vi "Measurement UI.vi"() -> ()   [LabVIEW 2020, in "Waveform Measurement.lvlib"]
uses:
  Waveform Measurement.lvlib
  <vilib>/gRPC/Generated APIs/ni/protobuf/types/RPC Messages/ni_protobuf_types_DoubleAnalogWaveform_Flat.ctl
  <vilib>/gRPC/Generated APIs/ni/protobuf/types/RPC Messages/ni_protobuf_types_PrecisionTimestamp_Flat.ctl
  <vilib>/gRPC/Generated APIs/ni/protobuf/types/RPC Messages/ni_protobuf_types_DoubleAnalogWaveform_AttributesEntry_Flat.ctl
  <vilib>/gRPC/Generated APIs/ni/protobuf/types/RPC Messages/ni_protobuf_types_WaveformAttributeValue_Flat.ctl
  <vilib>/gRPC/Extensions/Extensions.lvlib
  <vilib>/gRPC/Generated APIs/ni/protobuf/types/ni.protobuf.types.lvlib
panel:
  in  "Signal Type":T1(ring)=enum."Sine"
  out "Waveform":T2
  out "Waveform Graph":waveform(dbl)(graph)
  in  "Offset":dbl
  in  "Sample Rate":u32=1000
  in  "Frequency":dbl=10.0
  in  "Amplitude":dbl=5.0
  in  "Number of Samples":u32=1000
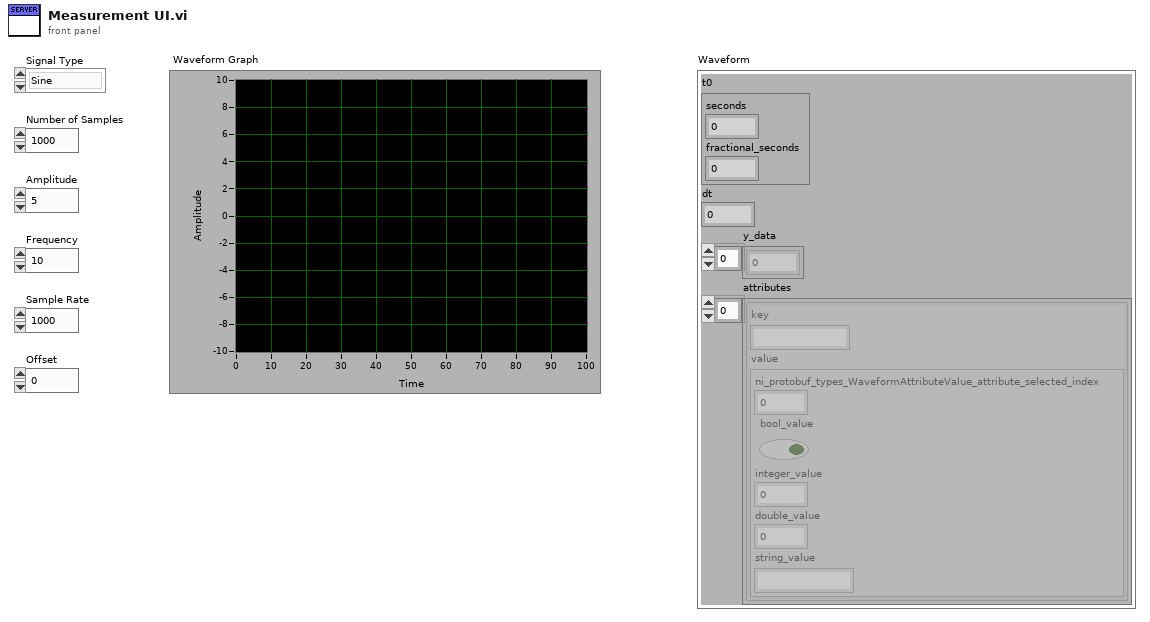
[diagram p1: front panel]
types:
  T1 = enum32{"None", "Sine", "Square", "Triangle", "Sawtooth"}
  T2 = typedef "ni.protobuf.types.lvlib/ni_protobuf_types_DoubleAnalogWaveform_Flat.ctl" = cluster{"t0":T3, "dt":dbl, "y_data":dbl[], "attributes":T4[]}
  T3 = typedef "ni.protobuf.types.lvlib/ni_protobuf_types_PrecisionTimestamp_Flat.ctl" = cluster{"seconds":i64, "fractional_seconds":u64}
  T4 = typedef "ni.protobuf.types.lvlib/ni_protobuf_types_DoubleAnalogWaveform_AttributesEntry_Flat.ctl" = cluster{"key":string, "value":T5}
  T5 = typedef "ni.protobuf.types.lvlib/ni_protobuf_types_WaveformAttributeValue_Flat.ctl" = cluster{"ni_protobuf_types_WaveformAttributeValue_attribute_selected_index":i32, "bool_value":bool, "integer_value":i32, "double_value":dbl, "string_value":string}
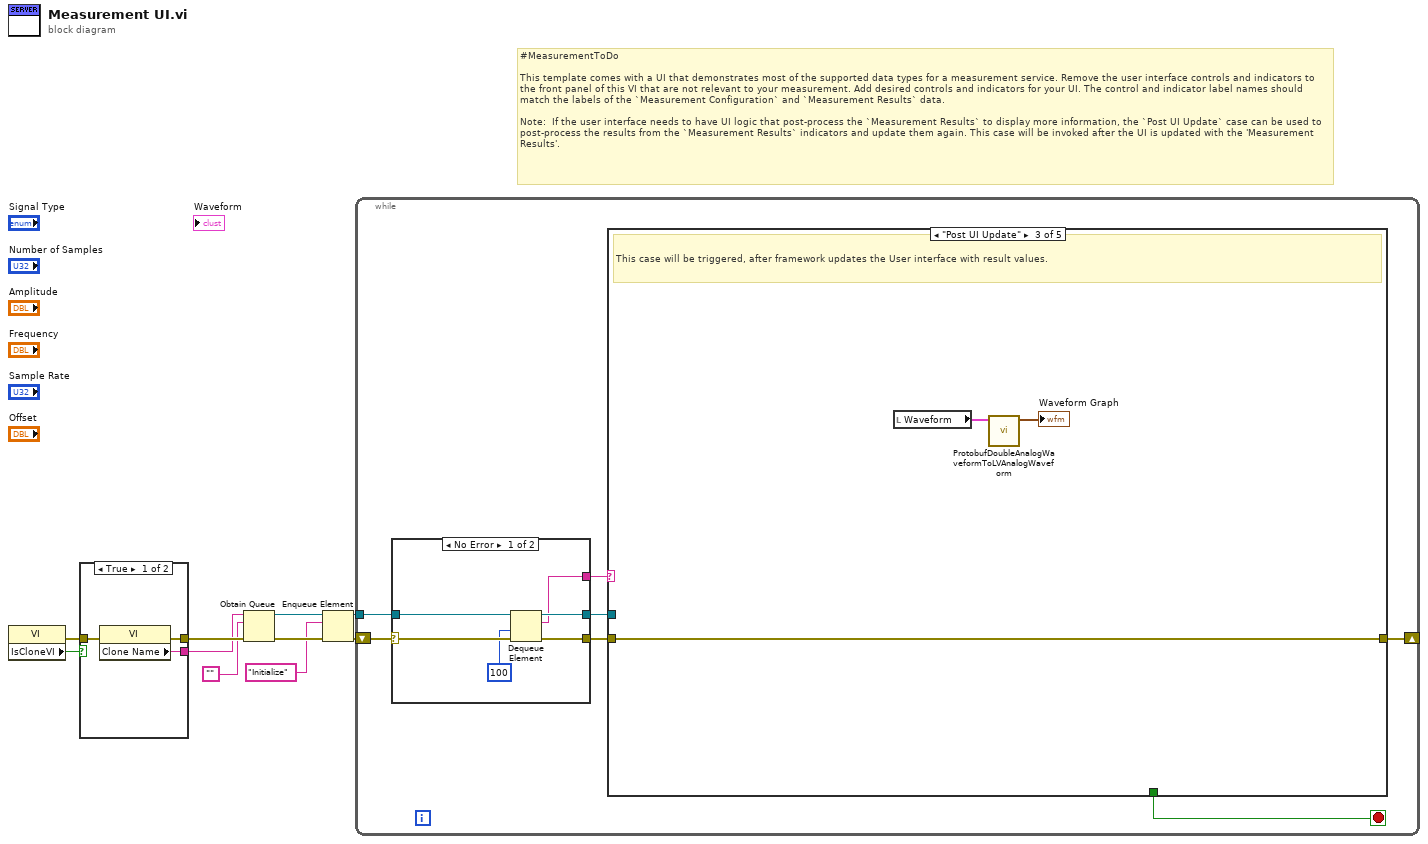
[diagram p0: block diagram]
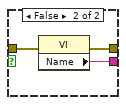
[diagram p2: hidden frame]
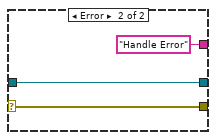
[diagram p3: hidden frame]
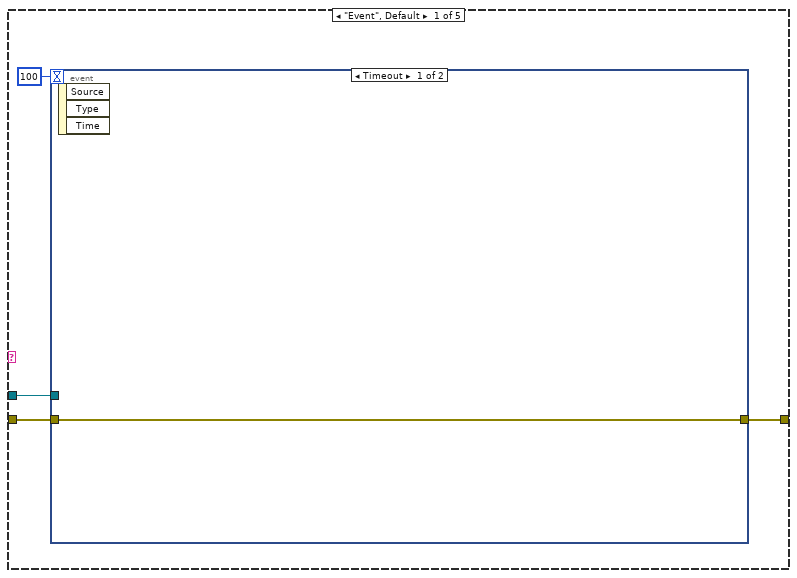
[diagram p4: hidden frame]
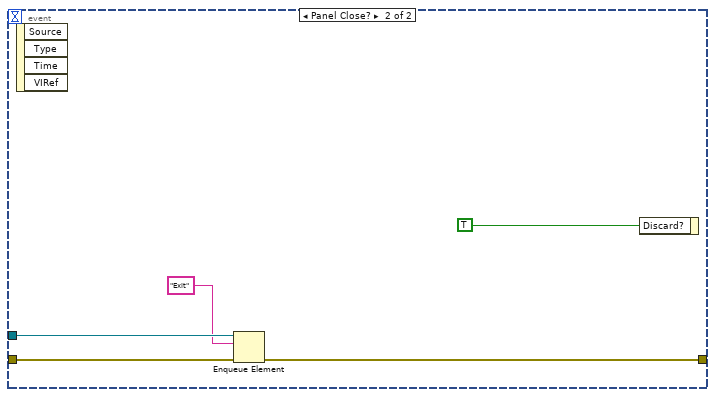
[diagram p5: hidden frame]
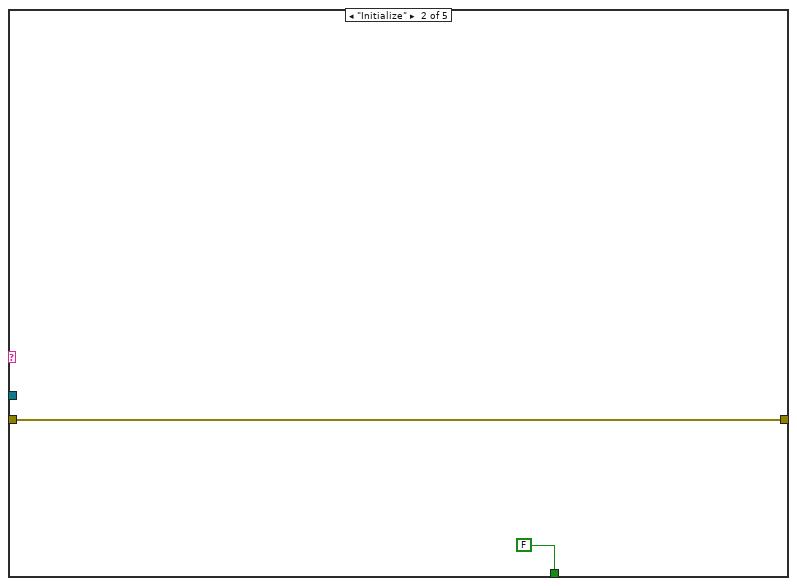
[diagram p6: hidden frame]
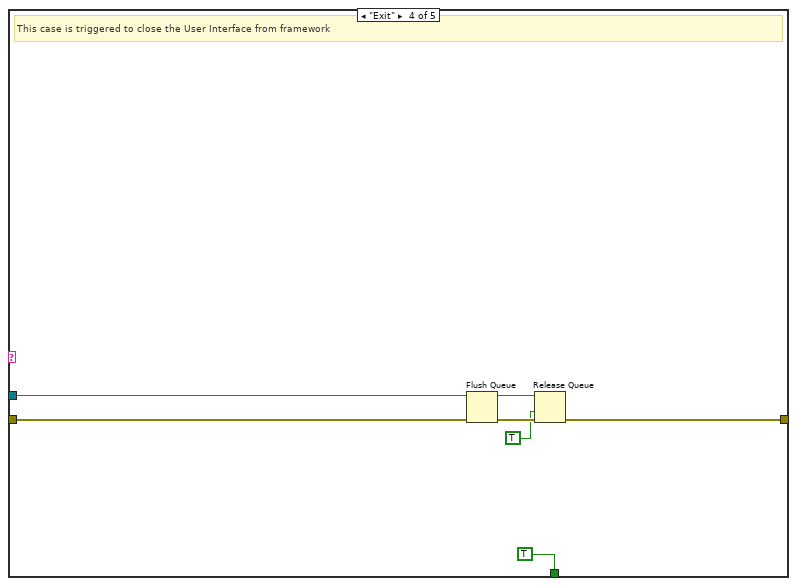
[diagram p7: hidden frame]
diagram:
  # "#MeasurementToDo  \n\nThis template comes with a UI that demonstrates most of the supported data types for a measurement service. Remove the user interface controls and indicators to the front panel of this VI that are not relevant to your measurement. Add desired controls and indicators for your UI. The control and indicator label names should match the labels of the `Measurement Configuration` and `Measurement Results` data.\n\nNote:  If the user interface needs to have UI logic that post-process the `Measurement Results` to display more information, the `Post UI Update` case can be used to post-process the results from the `Measurement Results` indicators and update them again. This case will be invoked after the UI is updated with the 'Measurement Results'."
  n1 = property class="VI"() -> (error out=w1:errorcluster, "IsCloneVI"=w2:bool)  [unwired: 2 in, 1 out]
  n2 = case shown="True" w2 {
    tunnel: [w13 w16] -> w10
    tunnel: [w12 w15] -> w9
    tunnel: w1 -> [w11 w14]
    frame True {
      n3 = property class="VI"(error in=w11) -> (error out=w13:errorcluster, "Clone Name"=w12:string)  [unwired: 1 in, 1 out]
    }
    frame False {
      n4 = property class="VI"(error in=w14) -> (error out=w16:errorcluster, "Name"=w15:string)  [unwired: 1 in, 1 out]
    }
  }
  n5 = Obtain Queue(name (unnamed)=w9, element data type="", error in (no error)=w10) -> (queue out=w6:refnum<queue>, error out=w8:errorcluster)  [unwired: 2 in, 1 out]
  n6 = Enqueue Element(queue=w6, element="Initialize", error in (no error)=w8) -> (queue out=w5:refnum<queue>, error out=w7:errorcluster)  [unwired: 1 in, 1 out]
  n7 = while {
    shift-right: [w18] -> _
    shift-left: w7 -> [w23]
    tunnel: w5 -> [w21]
    stop <- w17 stop-if-true
    n8 = case shown="No Error" w23 {
      selector: w23 -> [w29 w32]
      tunnel: [w28 w32] -> w22
      tunnel: w21 -> [w27 w31]
      tunnel: [w26 w31] -> w20
      tunnel: [w25 "Handle Error"] -> w19
      frame No Error {
        n9 = Dequeue Element(queue=w27, timeout in ms (-1)=100, error in (no error)=w29) -> (queue out=w26:refnum<queue>, element=w25:string, error out=w28:errorcluster)  [unwired: 1 out]
      }
      frame Error {
      }
    }
    n10 = case shown="\"Post UI Update\"" w19 {
      tunnel: w22 -> [w35 w44 w47 w54 w55]
      tunnel: w20 -> [w33 _ _ w52 _]
      tunnel: [w36 w44 w47 w49 w55] -> w18
      tunnel: [_ FALSE _ TRUE _] -> w17
      frame "Event", Default {
        n11 = event shown="[0] Timeout" {
          selector: _ -> [_ _]
          dyn-events: _ -> [_ _]
          timeout: 100 -> [_ _]
          tunnel: [w37 w40] -> w36
          tunnel: w35 -> [w37 w41]
          tunnel: w33 -> [_ w39]
          event Timeout {
            n12 = event-data() -> ()  [unwired: 1 in, 3 out]
          }
          event Panel Close? {
            n13 = event-data() -> ()  [unwired: 1 in, 4 out]
            n14 = Enqueue Element(queue=w39, element="Exit", error in (no error)=w41) -> (error out=w40:errorcluster)  [unwired: 1 in, 2 out]
            n15 = event-data("Discard?"=TRUE) -> ()  [unwired: 1 in, 1 out]
          }
        }
      }
      frame "Initialize" {
      }
      frame "Post UI Update" {
        # "This case will be triggered, after framework updates the User interface with result values."
        n16 = local read "Waveform"() -> (w46:T2)
        n17 = call <vilib>:"ProtobufDoubleAnalogWaveformToLVAnalogWaveform.vi"("ni_protobuf_types_DoubleAnalogWaveform_Flat"=w46) -> ("Waveform"=→"Waveform Graph":waveform(dbl))  [unwired: 9 in, 1 out]
      }
      frame "Exit" {
        # "This case is triggered to close the User Interface from framework"
        n18 = Flush Queue(queue=w52, error in (no error)=w54) -> (queue out=w51:refnum<queue>, error out=w50:errorcluster)  [unwired: 1 out]
        n19 = Release Queue(queue=w51, force destroy? (F)=TRUE, error in (no error)=w50) -> (error out=w49:errorcluster)  [unwired: 2 out]
      }
      frame "Handle Error" {
      }
    }
  }
